vi "Teleop.vi"(10 "Match Info":T1={"Autonomous Elapsed Seconds"=0.0, "TeleOp Elapsed Seconds"=0.0, "Disabled Elapsed Seconds"=0.0, "Visited Autonomous"=FALSE, "Visited TeleOp"=FALSE, "Visited Disabled"=FALSE, "Autonomous Settings"={"Autonomous Style"=enum."Independent", "VI Refnum"=refnum}}, 11 "Call Context":T2) -> ()   [LabVIEW 2014]
doc: "This VI is called for each TeleOp packet received from the DS where the robot is not disabled. It is often used to read from the joysticks and update I/O or to update setpoints for timed control loops. It should complete and return within 20 milliseconds or it may miss DS packets."
uses:
  <vilib>/Rock Robotics/WPI/DriverStation/WPI_DriverStationDerivedRobotMode.ctl
  <vilib>/Rock Robotics/WPI/DriverStation/WPI_DriverStationMatch Info.ctl
  Robot Global Data.vi
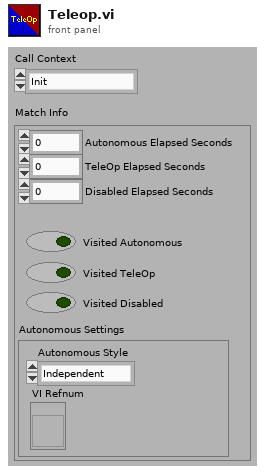
[diagram p1: front panel]
types:
  T1 = typedef "WPI_DriverStationMatch Info.ctl" = cluster{"Autonomous Elapsed Seconds":dbl, "TeleOp Elapsed Seconds":dbl, "Disabled Elapsed Seconds":dbl, "Visited Autonomous":bool, "Visited TeleOp":bool, "Visited Disabled":bool, "Autonomous Settings":cluster{"Autonomous Style":enum16{"Iterative", "Independent"}, "VI Refnum":refnum<vi>}}
  T2 = typedef "WPI_DriverStationDerivedRobotMode.ctl" = enum16{"Init", "Execute", "Stop"}
  T3 = cluster{"Left Power":dbl, "Right Power":dbl, "Shooter State":enum16{"Nothing", "Fire", "Load"}, "Loader State":enum16{"Loader Up", "Loader Down", "Ball In Possesion"}, "Auto Time":dbl, "Tele Time":dbl, "Driver":dbl, "Not Allowed":bool, "Right Speed":dbl, "Left Speed":dbl}
  T4 = enum16{"Nothing", "Load", "Lock", "Pass", "Grab", "Loader Down", "Shoot", "Auto Start", "Tele Start"}
  T5 = cluster{"Axes":cluster{"Triggers":dbl, "Right Stick Y":dbl, "Left Stick Y":dbl, "D-Pad":dbl, "Right Stick X":dbl, "Left Stick X":dbl}, "Buttons":cluster{"Left Bumper":bool, "Right Bumper":bool, "Y":bool, "A":bool, "X":bool, "B":bool, "Back":bool, "Start":bool, "Left Joystick":bool, "Right Joystick":bool}}
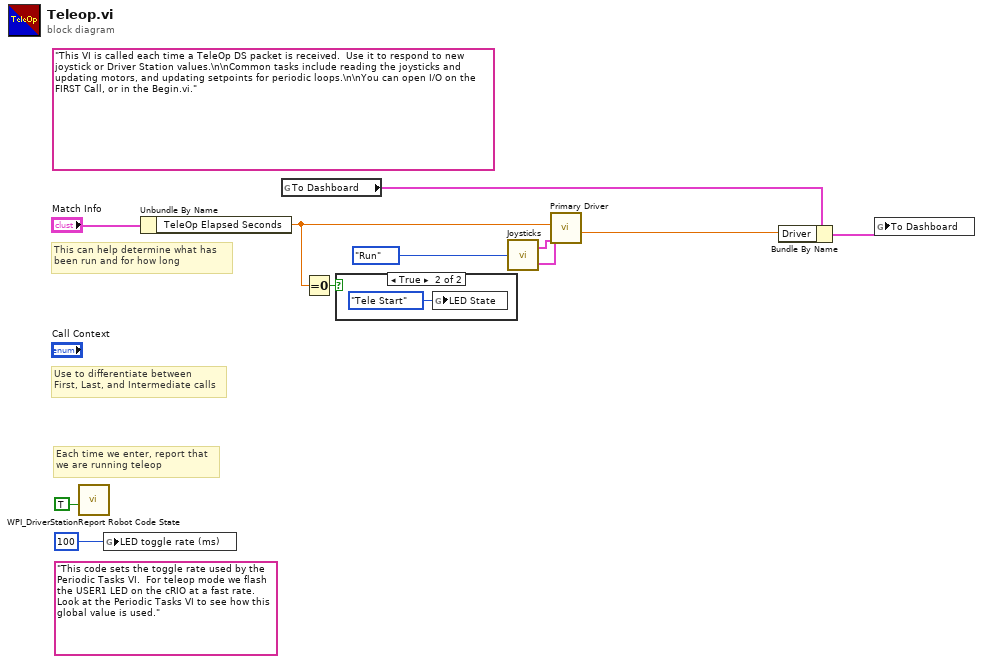
[diagram p0: block diagram]
diagram:
  (unwired) "This code sets the toggle rate used by the Periodic Tasks VI.  For teleop mode we flash the USER1 LED on the cRIO at a fast rate.  Look at the Periodic Tasks VI to see how this global value is used."
  (unwired) "This VI is called each time a TeleOp DS packet is received.  Use it to respond to new joystick or Driver Station values.\n\nCommon tasks include reading the joysticks and updating motors, and updating setpoints for periodic loops.\n\nYou can open I/O on the FIRST Call, or in the Begin.vi."
  # "Each time we enter, report that\nwe are running teleop"
  # "Use to differentiate between\nFirst, Last, and Intermediate calls"
  # "This can help determine what has\nbeen run and for how long"
  n1 = call <vilib>:"WPI_DriverStationReport Robot Code State.vi"("TeleOp"=TRUE ("Autonomous")) -> ()  [unwired: 10 in, 1 out]
  n2 = global write "Robot Global Data.vi" "LED toggle rate (ms)"(u32 100 ("LED ms toggle rate")) -> ()
  n3 = Unbundle By Name("Match Info") -> ("TeleOp Elapsed Seconds"=w4:dbl)
  n4 = global read "Robot Global Data.vi" "To Dashboard"() -> (w6:T3)
  n5 = Equal To 0?(x=w4) -> (x = 0?=w3:bool)
  n6 = case shown="True" w3 {
    frame False {
    }
    frame True {
      n7 = global write "Robot Global Data.vi" "LED State"(T4."Tele Start" ("LED State")) -> ()
    }
  }
  n8 = call "Joysticks.vi"("Enum"=enum16{"Start", "Run", "End"}."Run") -> ("Primary Driver"=w7:T5, "Secondary Driver"=w2:T5)
  n9 = call "Primary Driver.vi"("Primary Driver"=w7, "Secondary Driver"=w2, "Teleop Seconds"=w4) -> ("Driver"=w1:dbl)  [unwired: 6 in]
  n10 = Bundle By Name(cluster=w6, "Driver"=w1) -> (w5:T3)
  n11 = global write "Robot Global Data.vi" "To Dashboard"(w5) -> ()
